vi "Setup Arcadia_lv2013.vi"(11 "error in (no error)":errorcluster) -> (2 "LabVIEW Versions Present":string[](array[string]))   [LabVIEW 2014]
uses:
  <vilib>/nisyscfg/Get Installed Components.vi
  <vilib>/nisyscfg/Close (System).vi
  <vilib>/nisyscfg/nisyscfg.lvlib
panel:
  out "?":u8(slide) scale=0.0..100.0
  out "error out":errorcluster
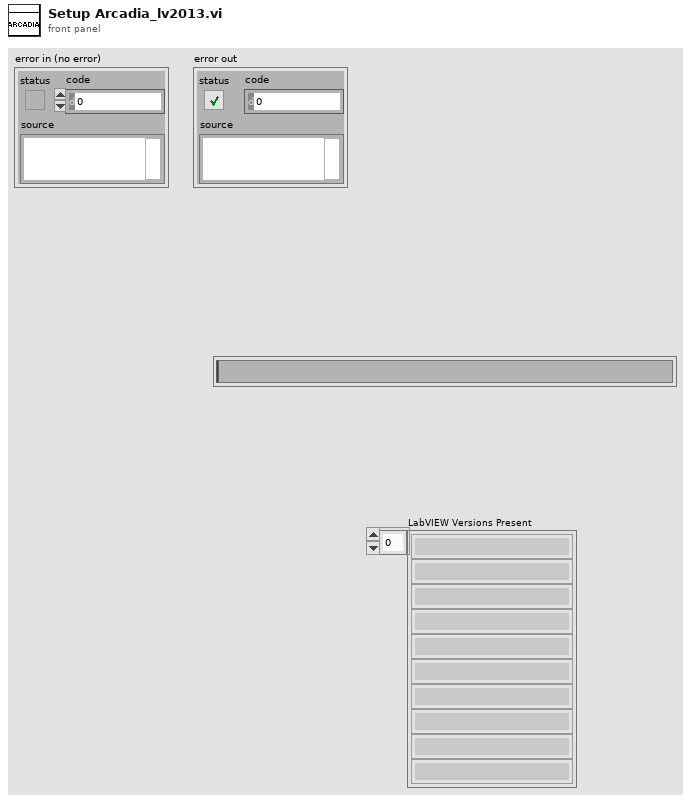
[diagram p1: front panel]
types:
  T1 = typedef "nisyscfg.lvlib/Software 1.2.ctl" = cluster{"title":string, "description":string, "ID":string, "version":string, "component type":T2}
  T2 = typedef "nisyscfg.lvlib/Component Type.ctl" = u32
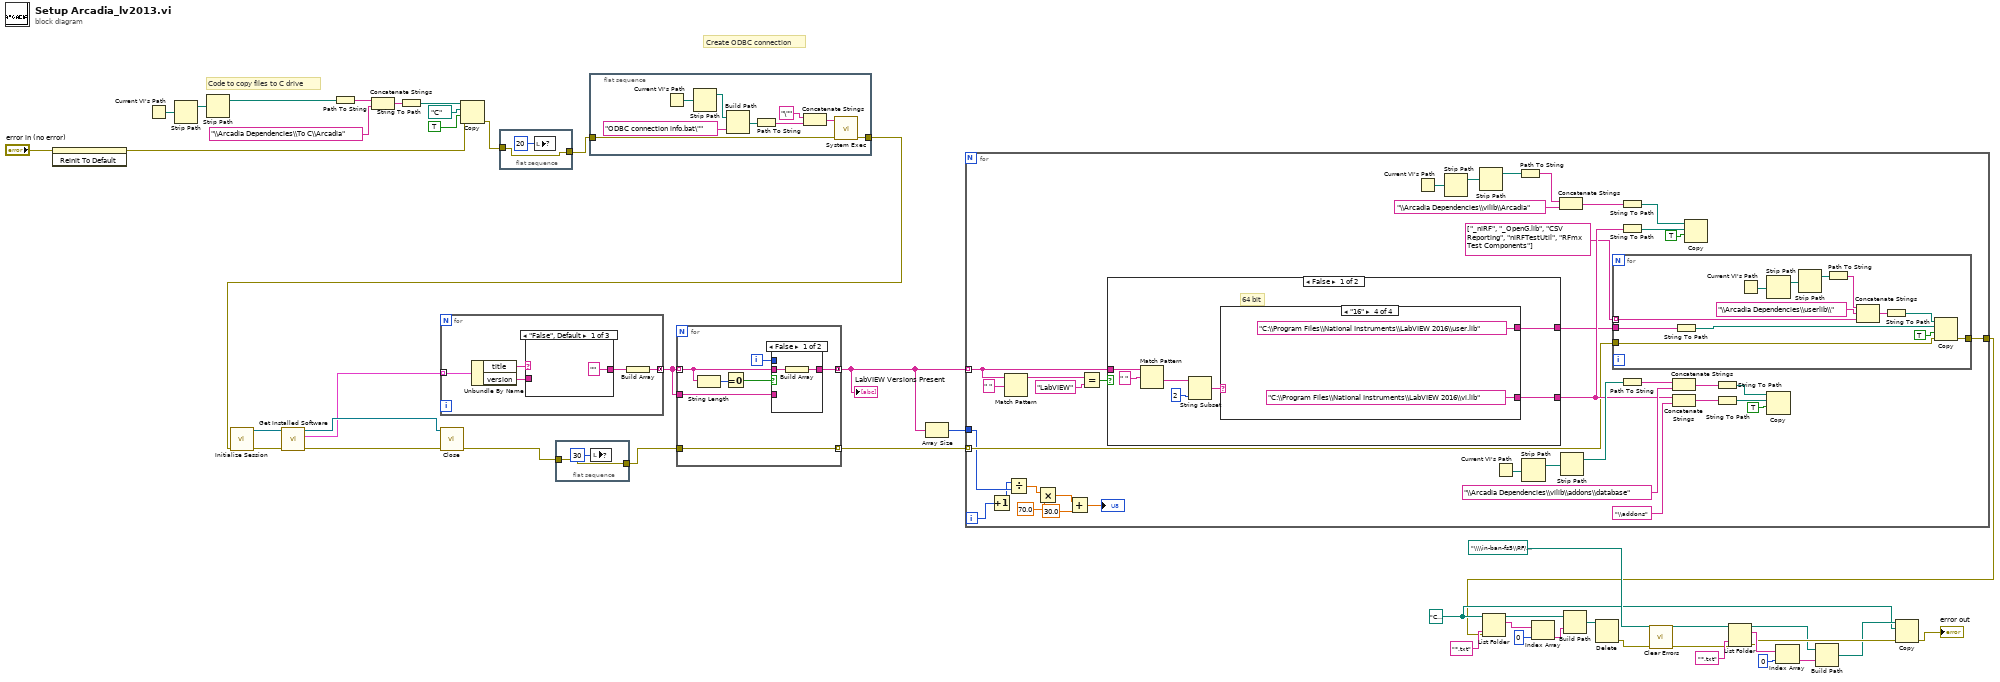
[diagram p0: block diagram]
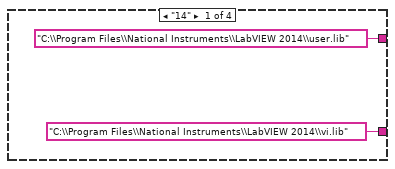
[diagram p2: hidden frame]
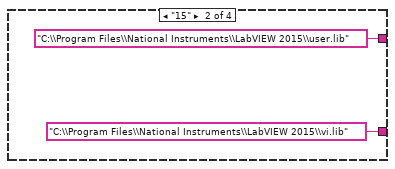
[diagram p3: hidden frame]
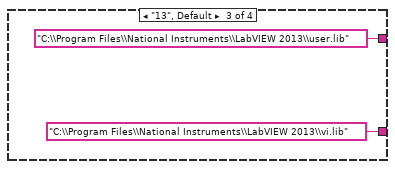
[diagram p4: hidden frame]
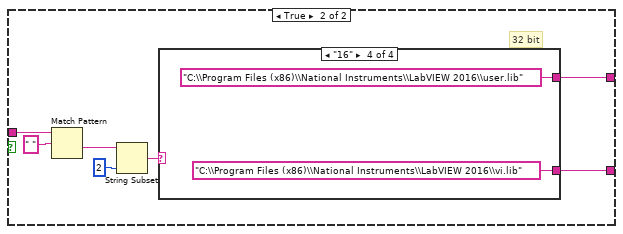
[diagram p5: hidden frame]
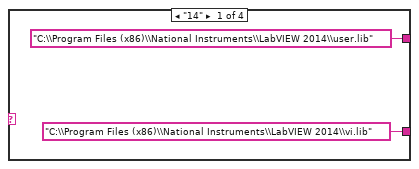
[diagram p6: hidden frame]
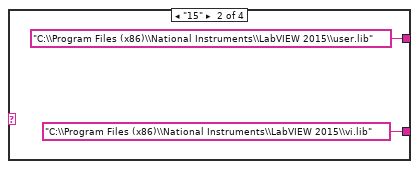
[diagram p7: hidden frame]
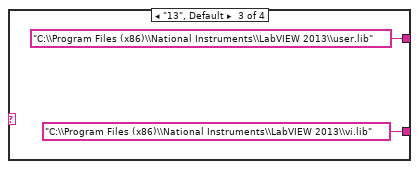
[diagram p8: hidden frame]
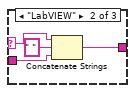
[diagram p10: hidden frame]
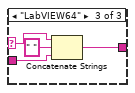
[diagram p11: hidden frame]
diagram:
  w5 = path "C:/Arcadia" ("path")
  # "Create ODBC connection"
  # "Code to copy files to C drive"
  n1 = invoke class="Slide (strict)" method="Reinit To Default"(error in="error in (no error)") -> (error out=w25:errorcluster)  [unwired: 2 in, 2 out]
  n2 = Current VI's Path() -> (path=w32:path)
  n3 = Strip Path(path=w32) -> (stripped path=w35:path)  [unwired: 1 out]
  n4 = Strip Path(path=w35) -> (stripped path=w36:path)  [unwired: 1 out]
  n5 = call <vilib>:"Initialize Session.vi"("error in (no error)"=w28) -> ("error out"=w43:errorcluster, "Session out"=w44:refnum<k21>)  [unwired: 9 in]
  n6 = call-poly <vilib>:"Get Installed Software.vi"("error in (no error)"=w43, "Session in"=w44) -> ("error out"=w42:errorcluster, "Software Components"=w40:T1[], "Session out"=w41:refnum<k21>)  [unwired: 7 in]
  n7 = Path To String(path=w36) -> (string=w33:string)
  n8 = Concatenate Strings(w33, "\\Arcadia Dependencies\\To C\\Arcadia" ("string")) -> (w31:string)
  n9 = String To Path(string=w31) -> (path=w30:path)
  n10 = for {
    tunnel: w40 -> [w49] mode=indexing
    tunnel: [w45] -> w39 mode=concatenating
    n11 = Unbundle By Name(w49) -> ("title"=w47:string, "version"=w48:string)
    n12 = case shown="\"False\", Default" w47 {
      selector: w47 -> [_ w54 w56]
      tunnel: w48 -> [_ w52 w57]
      tunnel: ["" w51 w55] -> w46
      frame "False", Default {
      }
      frame "LabVIEW" {
        n13 = Concatenate Strings(w54, " " ("string"), w52) -> (w51:string)
      }
      frame "LabVIEW64" {
        n14 = Concatenate Strings(w56, " " ("string"), w57) -> (w55:string)
      }
    }
    n15 = Build Array(w46) -> (w45:string[])
  }
  n16 = call-poly <vilib>:"Close.vi"("error in (no error)"=w42, "Session in"=w41) -> ("error out"=w21:errorcluster)  [unwired: 9 in]
  n17 = Copy(8:w25, 9:TRUE ("overwrite (F)"), 10:path "C:/" ("target path (use dialog)"), 11:w30) -> (0:w23:errorcluster)  [unwired: 1 in, 2 out]
  n18 = flat-sequence {
    tunnel: w23 -> [w59]
    tunnel: [w59] -> w22
    frame #0 {
      n19 = local write item#3(u8 20) -> ()
    }
  }
  n20 = flat-sequence {
    tunnel: [w61] -> _
    tunnel: [w61] -> w20
    tunnel: w21 -> [w61]
    frame #0 {
      n21 = local write item#3(u8 30) -> ()
    }
  }
  n22 = flat-sequence {
    tunnel: w22 -> [w64]
    tunnel: [w63] -> w28
    frame #0 {
      n23 = Current VI's Path() -> (path=w71:path)
      n24 = Strip Path(path=w71) -> (stripped path=w70:path)  [unwired: 1 out]
      n25 = Build Path(base path=w70, name or relative path="ODBC connection info.bat\"") -> (appended path=w68:path)
      n26 = Path To String(path=w68) -> (string=w67:string)
      n27 = Concatenate Strings("\"" ("string"), w67) -> (w65:string)
      n28 = call <vilib>:"System Exec.vi"("error in (no error)"=w64, "command line"=w65) -> ("error out"=w63:errorcluster)  [unwired: 6 in, 3 out]
    }
  }
  n29 = for {
    tunnel: w39 -> [w74] mode=indexing
    tunnel: w39 -> [w75]
    tunnel: [w73] -> w27 mode=concatenating
    tunnel: w20 -> [w72]
    tunnel: [w72] -> w29 mode=indexing
    i -> [w76]
    n30 = String Length(string=w74) -> (length=w78:i32)
    n31 = Equal To 0?(x=w78) -> (x = 0?=w77:bool)
    n32 = case shown="False" w77 {
      tunnel: w76 -> [_ _]
      tunnel: w75 -> [_ _]
      tunnel: w74 -> [w80 _]
      tunnel: [w79 _] -> w73
      frame False {
        n33 = Build Array(w80) -> (w79:string[])
      }
      frame True {
      }
    }
  }
  "LabVIEW Versions Present" <- w27
  n34 = Array Size(array=w27) -> (size(s)=w26:i32)
  n35 = for {
    tunnel: w27 -> [w114] mode=indexing
    tunnel: [w90] -> w2
    tunnel: w29 -> [w89] mode=indexing
    tunnel: w26 -> [w88]
    i -> [w82]
    n36 = Increment(x=w82) -> (x+1=w81:i32)
    n37 = Match Pattern(string=w114, regular expression=" ") -> (before substring=w115:string)  [unwired: 1 in, 3 out]
    n38 = Divide(x=w81, y=w88) -> (x/y=w87:dbl)
    n39 = Multiply(x=w87, y=70.0 ("x")) -> (x*y=w85:dbl)
    n40 = Add(x=w85, y=30.0) -> (x+y=→"?":dbl)
    n41 = Equal?(x=w115, y="LabVIEW") -> (x = y?=w116:bool)
    n42 = case shown="False" w116 {
      tunnel: w114 -> [w137 w152]
      tunnel: [w133 w148] -> w95
      tunnel: [w132 w147] -> w91
      frame False {
        # "64 bit"
        n43 = Match Pattern(string=w137, regular expression=" ") -> (after substring=w136:string)  [unwired: 1 in, 3 out]
        n44 = String Subset(string=w136, length (rest)=2 ("length (rest)")) -> (substring=w134:string)  [unwired: 1 in]
        n45 = case shown="\"16\"" w134 {
          tunnel: ["C:\\Program Files\\National Instruments\\LabVIEW 2014\\vi.lib" "C:\\Program Files\\National Instruments\\LabVIEW 2015\\vi.lib" "C:\\Program Files\\National Instruments\\LabVIEW 2013\\vi.lib" "C:\\Program Files\\National Instruments\\LabVIEW 2016\\vi.lib"] -> w133
          tunnel: ["C:\\Program Files\\National Instruments\\LabVIEW 2014\\user.lib" "C:\\Program Files\\National Instruments\\LabVIEW 2015\\user.lib" "C:\\Program Files\\National Instruments\\LabVIEW 2013\\user.lib" "C:\\Program Files\\National Instruments\\LabVIEW 2016\\user.lib"] -> w132
          frame "14" {
          }
          frame "15" {
          }
          frame "13", Default {
          }
          frame "16" {
          }
        }
      }
      frame True {
        # "32 bit"
        n46 = Match Pattern(string=w152, regular expression=" ") -> (after substring=w150:string)  [unwired: 1 in, 3 out]
        n47 = String Subset(string=w150, length (rest)=2 ("length (rest)")) -> (substring=w149:string)  [unwired: 1 in]
        n48 = case shown="\"16\"" w149 {
          tunnel: ["C:\\Program Files (x86)\\National Instruments\\LabVIEW 2014\\vi.lib" "C:\\Program Files (x86)\\National Instruments\\LabVIEW 2015\\vi.lib" "C:\\Program Files (x86)\\National Instruments\\LabVIEW 2013\\vi.lib" "C:\\Program Files (x86)\\National Instruments\\LabVIEW 2016\\vi.lib"] -> w148
          tunnel: ["C:\\Program Files (x86)\\National Instruments\\LabVIEW 2014\\user.lib" "C:\\Program Files (x86)\\National Instruments\\LabVIEW 2015\\user.lib" "C:\\Program Files (x86)\\National Instruments\\LabVIEW 2013\\user.lib" "C:\\Program Files (x86)\\National Instruments\\LabVIEW 2016\\user.lib"] -> w147
          frame "14" {
          }
          frame "15" {
          }
          frame "13", Default {
          }
          frame "16" {
          }
        }
      }
    }
    n49 = Current VI's Path() -> (path=w108:path)
    n50 = Strip Path(path=w108) -> (stripped path=w111:path)  [unwired: 1 out]
    n51 = Strip Path(path=w111) -> (stripped path=w112:path)  [unwired: 1 out]
    n52 = Current VI's Path() -> (path=w101:path)
    n53 = Path To String(path=w112) -> (string=w109:string)
    n54 = Strip Path(path=w101) -> (stripped path=w98:path)  [unwired: 1 out]
    n55 = Concatenate Strings(w109, "\\Arcadia Dependencies\\vilib\\Arcadia" ("string")) -> (w107:string)
    n56 = Strip Path(path=w98) -> (stripped path=w97:path)  [unwired: 1 out]
    n57 = for {
      tunnel: string[] ["_niRF", "_OpenG.lib", "CSV Reporting", "niRFTestUtil", "RFmx Test Components"] -> [w122] mode=indexing
      tunnel: w91 -> [w121]
      tunnel: [w120] -> w90
      tunnel: w89 -> [w119]
      n58 = String To Path(string=w121) -> (path=w123:path)
      n59 = Current VI's Path() -> (path=w131:path)
      n60 = Strip Path(path=w131) -> (stripped path=w128:path)  [unwired: 1 out]
      n61 = Strip Path(path=w128) -> (stripped path=w127:path)  [unwired: 1 out]
      n62 = Path To String(path=w127) -> (string=w130:string)
      n63 = Concatenate Strings(w130, "\\Arcadia Dependencies\\userlib\\" ("string"), w122) -> (w125:string)
      n64 = String To Path(string=w125) -> (path=w124:path)
      n65 = Copy(8:w119, 9:TRUE ("overwrite (F)"), 10:w123, 11:w124) -> (0:w120:errorcluster)  [unwired: 1 in, 2 out]
    }
    n66 = String To Path(string=w107) -> (path=w106:path)
    n67 = String To Path(string=w95) -> (path=w105:path)
    n68 = Path To String(path=w97) -> (string=w100:string)
    n69 = Concatenate Strings(w100, "\\Arcadia Dependencies\\vilib\\addons\\database" ("string")) -> (w102:string)
    n70 = Concatenate Strings(w95, "\\addons" ("string")) -> (w93:string)
    n71 = Copy(9:TRUE ("overwrite (F)"), 10:w105, 11:w106) -> ()  [unwired: 2 in, 3 out]
    n72 = String To Path(string=w102) -> (path=w103:path)
    n73 = String To Path(string=w93) -> (path=w104:path)
    n74 = Copy(9:TRUE ("overwrite (F)"), 10:w104, 11:w103) -> ()  [unwired: 2 in, 3 out]
  }
  n75 = List Folder(path=w5, pattern="*.txt", error in=w2) -> (path out=w18:path, filenames=w17:string[])  [unwired: 1 in, 2 out]
  n76 = Index Array(array=w17, index=0) -> (element=w15:string)
  n77 = Build Path(base path=w18, name or relative path=w15) -> (appended path=w14:path)
  n78 = Delete(path (use dialog)=w14) -> (error out=w4:errorcluster)  [unwired: 4 in, 2 out]
  n79 = call <vilib>:"Clear Errors.vi"("error in (no error)"=w4) -> ("error out"=w3:errorcluster)  [unwired: 5 in, 1 out]
  n80 = List Folder(path=path "\\\\in-ban-fs5\\RF/Arcadia/Arcadia Dependencies", pattern="*.txt", error in=w3) -> (path out=w7:path, filenames=w10:string[], error out=w9:errorcluster)  [unwired: 1 in, 1 out]
  n81 = Index Array(array=w10, index=0) -> (element=w8:string)
  n82 = Build Path(base path=w7, name or relative path=w8) -> (appended path=w6:path)
  n83 = Copy(8:w9, 10:w5, 11:w6) -> (0:→"error out":errorcluster)  [unwired: 2 in, 2 out]
